vi "Get Parameter Value (single).vi"(6 "Clear Null":bool=TRUE, 10 "Parameter Name":string, 11 "JSON":string) -> (1 "Found":bool, 2 "Parameter Value":string, 3 "Remaining JSON":string, 4 "Null":bool)   [LabVIEW 2015, in "NI_Azure_JSON Parsing.lvlib"]
uses:
  NI_Azure_JSON Parsing.lvlib
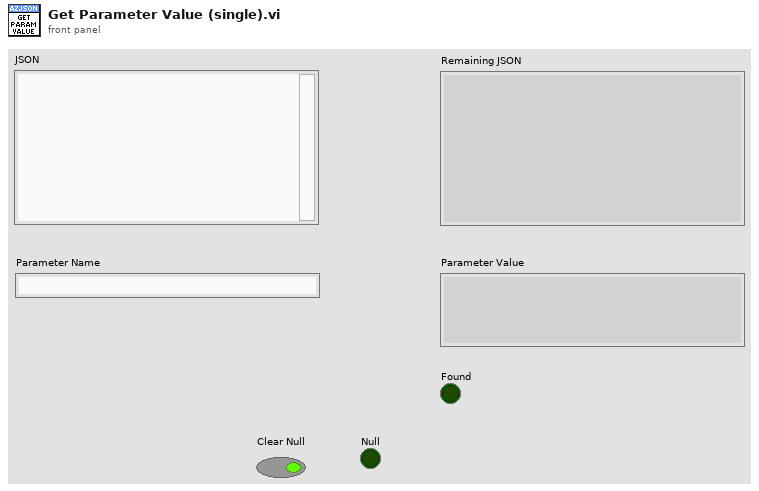
[diagram p1: front panel]
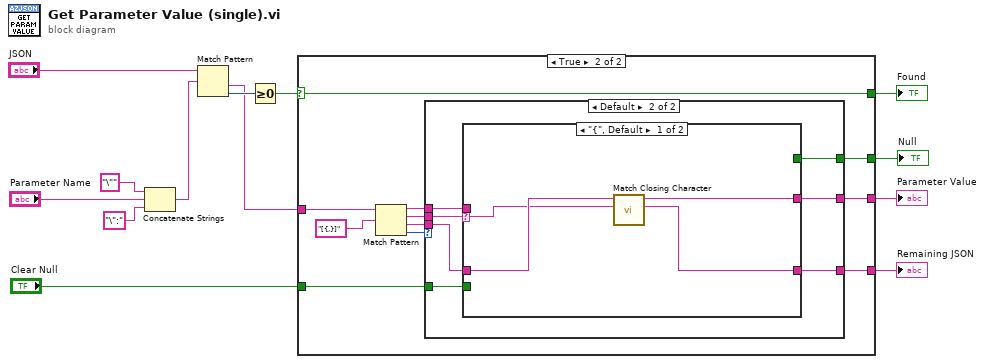
[diagram p0: block diagram]
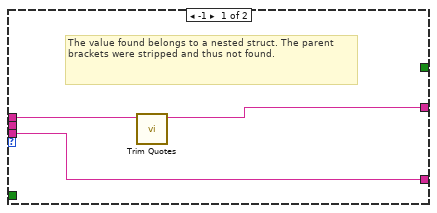
[diagram p3: hidden frame]
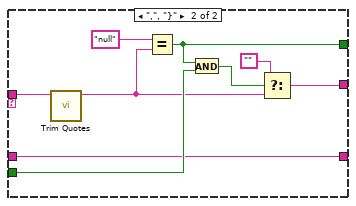
[diagram p4: hidden frame]
diagram:
  n1 = Concatenate Strings("\"" ("string"), "Parameter Name", "\":" ("string")) -> (w11:string)
  n2 = Match Pattern(string="JSON", regular expression=w11) -> (after substring=w3:string, offset past match=w8:i32)  [unwired: 1 in, 2 out]
  n3 = Greater Or Equal To 0?(x=w8) -> (x >= 0?=w2:bool)
  n4 = case shown="True" w2 {
    selector: w2 -> [_ w15]
    tunnel: "Clear Null" -> [_ w22]
    tunnel: [_ w21] -> w6
    tunnel: [_ w20] -> w5
    tunnel: [_ w18] -> w4
    tunnel: w3 -> [_ w16]
    tunnel: [_ w15] -> w1
    frame False {
    }
    frame True {
      n5 = Match Pattern(string=w16, regular expression="[{,}]") -> (before substring=w23:string, match substring=w19:string, after substring=w17:string, offset past match=w14:i32)  [unwired: 1 in]
      n6 = case shown="Default" w14 {
        tunnel: w23 -> [w27 w34]
        tunnel: w22 -> [_ w33]
        tunnel: [_ w32] -> w21
        tunnel: [w26 w31] -> w20
        tunnel: w19 -> [_ w30]
        tunnel: [w25 w29] -> w18
        tunnel: w17 -> [w25 w28]
        frame -1 {
          # "The value found belongs to a nested struct. The parent brackets were stripped and thus not found."
          n7 = call "Trim Quotes.vi"("String"=w27) -> ("String without Quotes"=w26:string)  [unwired: 9 in, 1 out]
        }
        frame Default {
          n8 = case shown="\"{\", Default" w30 {
            selector: w30 -> [w35 _]
            tunnel: w34 -> [_ w47]
            tunnel: w33 -> [_ w45]
            tunnel: [_ w44] -> w32
            tunnel: [w37 w42] -> w31
            tunnel: [w36 w39] -> w29
            tunnel: w28 -> [w38 w39]
            frame "{", Default {
              n9 = call "Match Closing Character.vi"("Open character"=w35, "JSON"=w38) -> ("rest of JSON"=w36:string, "match"=w37:string)  [unwired: 7 in, 1 out]
            }
            frame ",", "}" {
              n10 = call "Trim Quotes.vi"("String"=w47) -> ("String without Quotes"=w43:string)  [unwired: 9 in, 1 out]
              n11 = Equal?(x="null", y=w43) -> (x = y?=w44:bool)
              n12 = And(x=w44, y=w45) -> (x .and. y?=w41:bool)
              n13 = Select(t="", s=w41, f=w43) -> (s? t:f=w42:string)
            }
          }
        }
      }
    }
  }
  "Parameter Value" <- w5
  "Remaining JSON" <- w4
  "Found" <- w1
  "Null" <- w6
